vi "Excel Report - Generate from Template.vi"() -> ()   [LabVIEW 2015]
doc: "This example shows how to generate a report from a template. The template contains a preformatted table and a preformatted graph which are updated with Append Table to Report.vi and Excel Update Graph.vi."
uses:
  <vilib>/Utility/NIReport.llb/Append Report Text (str wrap).vi
  <vilib>/Utility/NIReport.llb/Append Text Table to Report (wrap).vi
  <vilib>/Utility/NIReport.llb/NI_report.lvclass
  <vilib>/Utility/NIReport.llb/Excel/NI_Excel.lvclass
panel:
  in  "Protocol File Name":string="100"
  in  "Test operator":string="Operator's name"
  in  "Run Ended":string="100"
  in  "Run Started":string="70"
  in  "File Name":string="20"
  in  "Data":string[][](table)=[["100", "41.7", "38.5"], ["125", "41.7", "35.2"], ["160", "41.5", "37.5"], ["200", "42.3", "42.5"], ["250", "46.9", "46.8"], ["315", "51.9", "52.6"], ["400", "52.3", "46.7"], ["500  ", "46.5", "41.6"], ["630", "42.3", "35.9"], ["800", "41.1", "32.6"]]
  # "Overview: This example shows how to generate a report from a template using either the Excel Report Generation VIs or the MS Office Report Express VI.\nRequirements: Report Generation Toolkit, Microsoft Excel\nInstructions:\nRun the VI."
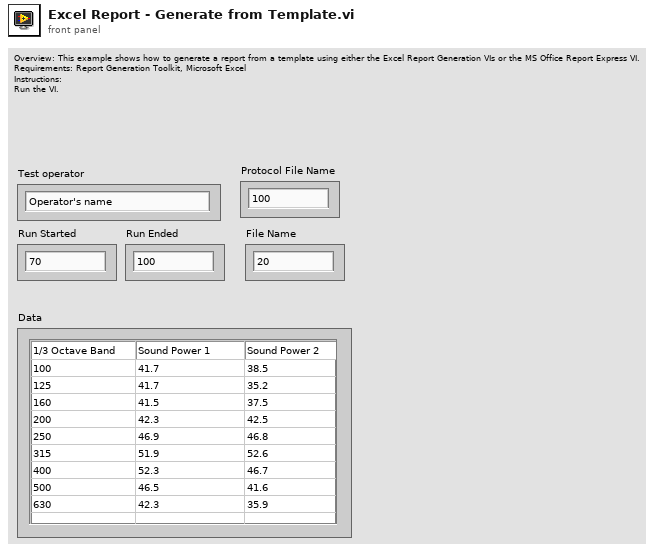
[diagram p1: front panel]
types:
  T1 = cluster{"position (Excel)":cluster{"row":i32, "column":i32}, "name (Excel)":string, "bookmark (Word)":string}
  T2 = enum16{"Standard Report", "HTML", "Word", "Excel"}
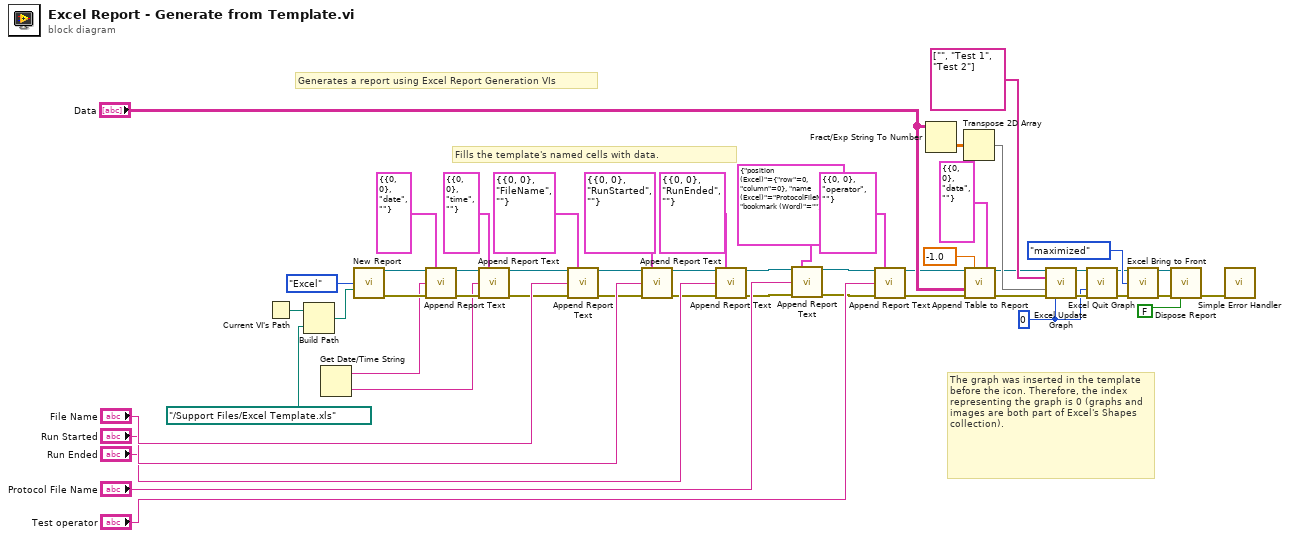
[diagram p0: block diagram]
diagram:
  w24 = i16 0 ("graph index")
  # "Fills the template's named cells with data."
  # "The graph was inserted in the template before the icon. Therefore, the index representing the graph is 0 (graphs and images are both part of Excel's Shapes collection)."
  # "Generates a report using Excel Report Generation VIs"
  n1 = Current VI's Path() -> (path=w7:path)
  n2 = Build Path(base path=w7, name or relative path=path "../Support Files/Excel Template.xls") -> (appended path=w32:path)
  n3 = Get Date/Time String() -> (date string=w8:string, time string=w9:string)  [unwired: 3 in]
  n4 = call <vilib>:"New Report.vi"("report type"=T2."Excel", "template (empty)"=w32) -> ("report out"=w38:refnum<class "NI_report.lvclass">, "error out"=w43:errorcluster)  [unwired: 12 in]
  n5 = call-poly <vilib>:"Append Report Text.vi"("report in"=w38, "MS Office parameters"=T1 {"position (Excel)"={"row"=0, "column"=0}, "name (Excel)"="date", "bookmark (Word)"=""}, "text"=w8, "error in (no error)"=w43) -> ("report out"=w37:refnum<class "NI_report.lvclass">, "error out"=w42:errorcluster)  [unwired: 8 in, 2 out]
  n6 = call-poly <vilib>:"Append Report Text.vi"("report in"=w37, "MS Office parameters"=T1 {"position (Excel)"={"row"=0, "column"=0}, "name (Excel)"="time", "bookmark (Word)"=""}, "text"=w9, "error in (no error)"=w42) -> ("report out"=w36:refnum<class "NI_report.lvclass">, "error out"=w41:errorcluster)  [unwired: 8 in, 2 out]
  n7 = call-poly <vilib>:"Append Report Text.vi"("report in"=w36, "MS Office parameters"=T1 {"position (Excel)"={"row"=0, "column"=0}, "name (Excel)"="FileName", "bookmark (Word)"=""}, "text"="File Name", "error in (no error)"=w41) -> ("report out"=w35:refnum<class "NI_report.lvclass">, "error out"=w40:errorcluster)  [unwired: 8 in, 2 out]
  n8 = call-poly <vilib>:"Append Report Text.vi"("report in"=w35, "MS Office parameters"=T1 {"position (Excel)"={"row"=0, "column"=0}, "name (Excel)"="RunStarted", "bookmark (Word)"=""}, "text"="Run Started", "error in (no error)"=w40) -> ("report out"=w34:refnum<class "NI_report.lvclass">, "error out"=w39:errorcluster)  [unwired: 8 in, 2 out]
  n9 = call-poly <vilib>:"Append Report Text.vi"("report in"=w34, "MS Office parameters"=T1 {"position (Excel)"={"row"=0, "column"=0}, "name (Excel)"="RunEnded", "bookmark (Word)"=""}, "text"="Run Ended", "error in (no error)"=w39) -> ("report out"=w3:refnum<class "NI_report.lvclass">, "error out"=w5:errorcluster)  [unwired: 8 in, 2 out]
  n10 = call-poly <vilib>:"Append Report Text.vi"("report in"=w3, "MS Office parameters"=T1 {"position (Excel)"={"row"=0, "column"=0}, "name (Excel)"="ProtocolFileName", "bookmark (Word)"=""}, "text"="Protocol File Name", "error in (no error)"=w5) -> ("report out"=w2:refnum<class "NI_report.lvclass">, "error out"=w4:errorcluster)  [unwired: 8 in, 2 out]
  n11 = call-poly <vilib>:"Append Report Text.vi"("report in"=w2, "MS Office parameters"=T1 {"position (Excel)"={"row"=0, "column"=0}, "name (Excel)"="operator", "bookmark (Word)"=""}, "text"="Test operator", "error in (no error)"=w4) -> ("report out"=w21:refnum<class "NI_report.lvclass">, "error out"=w20:errorcluster)  [unwired: 8 in, 2 out]
  n12 = Fract/Exp String To Number(string="Data") -> (number=w44:dbl[][])  [unwired: 3 in, 1 out]
  n13 = Transpose 2D Array(2D array=w44) -> (transposed array=w22:dbl[][])
  n14 = call-poly <vilib>:"Append Table to Report.vi"("report in"=w21, "column width (1)"=-1.0, "MS Office parameters"=T1 {"position (Excel)"={"row"=0, "column"=0}, "name (Excel)"="data", "bookmark (Word)"=""}, "text data"="Data", "error in (no error)"=w20) -> ("report out"=w19:refnum<class "NI_report.lvclass">, "error out"=w18:errorcluster)  [unwired: 7 in, 2 out]
  n15 = call <vilib>:"Excel Update Graph.vi"("report in"=w19, "row header"=string[] ["", "Test 1", "Test 2"], "graph data"=w22, "error in (no error)"=w18, "graph index (-1)"=w24) -> ("report out"=w26:refnum<class "NI_report.lvclass">, "error out"=w25:errorcluster)  [unwired: 9 in]
  n16 = call <vilib>:"Excel Quit Graph.vi"("report in"=w26, "graph index (-1)"=w24, "error in (no error)"=w25) -> ("report out"=w27:refnum<class "NI_report.lvclass">, "error out"=w28:errorcluster)  [unwired: 11 in]
  n17 = call <vilib>:"Excel Bring to Front.vi"("report in"=w27, "window state (maximized)"=enum16{"maximized", "minimized", "normal"}."maximized", "error in (no error)"=w28) -> ("report out"=w31:refnum<class "NI_report.lvclass">, "error out"=w30:errorcluster)  [unwired: 11 in]
  n18 = call-dynamic "Dispose Report.vi"("report in"=w31, "error in (no error)"=w30, "close report? (T)"=FALSE ("Close Report? (T)")) -> ("error out"=w48:errorcluster)  [unwired: 12 in]
  n19 = call <vilib>:"Simple Error Handler.vi"("error in (no error)"=w48) -> ()  [unwired: 4 in, 5 out]
